vi "Arm Loop.vi"(8 "error in (no error)":errorcluster) -> ()   [LabVIEW 2012]
uses:
  Robot Global Data.vi
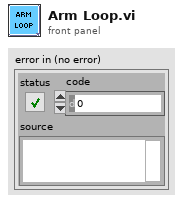
[diagram p1: front panel]
types:
  T1 = typedef "WPI_DriverStationRobotMode2.ctl" = enum16{"Autonomous Disabled", "Autonomous Enabled", "Teleop Disabled", "Teleop Enabled", "Timeout", "Finish", "Test Disabled", "Test Enabled"}
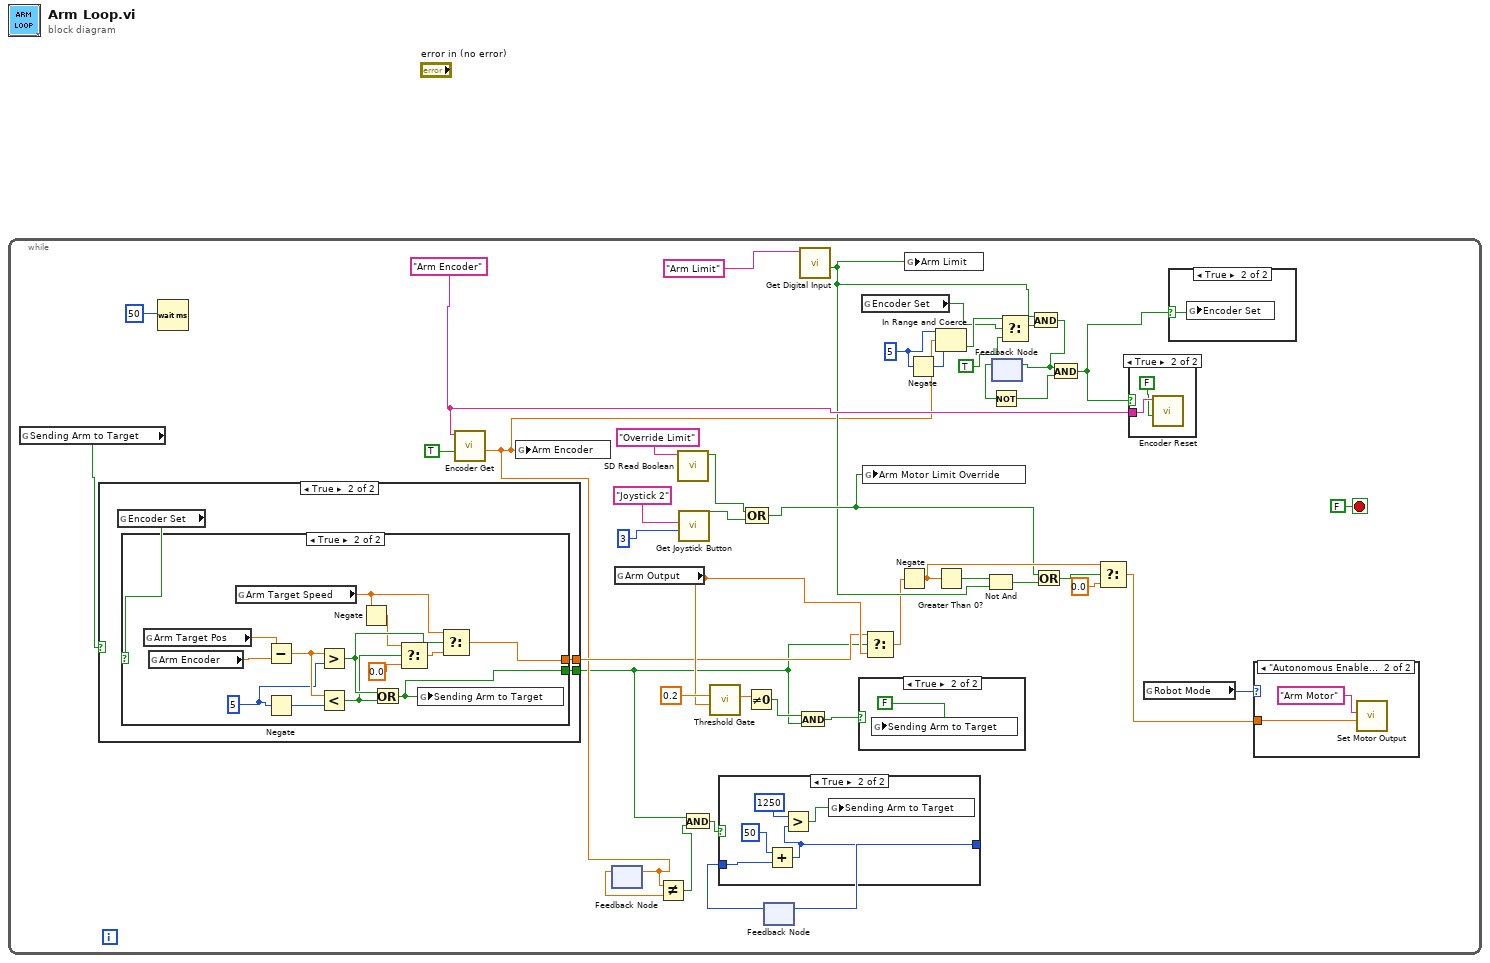
[diagram p0: block diagram]
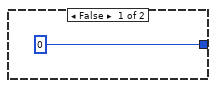
[diagram p2: hidden frame]
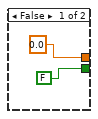
[diagram p5: hidden frame]
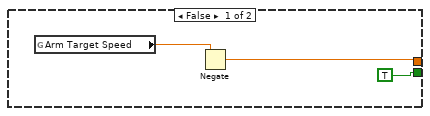
[diagram p6: hidden frame]
diagram:
  n1 = while {
    stop <- FALSE stop-if-true
    w26 = 5
    w29 = "Arm Encoder"
    n2 = global read "Robot Global Data.vi" "Sending Arm to Target"() -> (w16:bool)
    n3 = case shown="True" w16 {
      tunnel: [FALSE w57] -> w3
      tunnel: [0.0 w56] -> w12
      frame False {
      }
      frame True {
        n4 = global read "Robot Global Data.vi" "Encoder Set"() -> (w58:bool)
        n5 = case shown="True" w58 {
          tunnel: [TRUE w62] -> w57
          tunnel: [w60 w63] -> w56
          frame False {
            n6 = global read "Robot Global Data.vi" "Arm Target Speed"() -> (w61:dbl)
            n7 = Negate(x=w61) -> (-x=w60:dbl)
          }
          frame True {
            w66 = 5
            n8 = global read "Robot Global Data.vi" "Arm Target Pos"() -> (w67:dbl)
            n9 = global read "Robot Global Data.vi" "Arm Encoder"() -> (w68:dbl)
            n10 = global read "Robot Global Data.vi" "Arm Target Speed"() -> (w64:dbl)
            n11 = Subtract(x=w67, y=w68) -> (x-y=w74:dbl)
            n12 = Negate(x=w66) -> (-x=w73:i32)
            n13 = Greater?(x=w74, y=w66) -> (0:w71:bool)
            n14 = Less?(x=w74, y=w73) -> (x < y?=w69:bool)
            n15 = Negate(x=w64) -> (-x=w65:dbl)
            n16 = Or(x=w71, y=w69) -> (x .or. y?=w62:bool)
            n17 = Select(t=w65, s=w69, f=0.0) -> (s? t:f=w70:dbl)
            n18 = global write "Robot Global Data.vi" "Sending Arm to Target"(w62) -> ()
            n19 = Select(t=w64, s=w71, f=w70) -> (s? t:f=w63:dbl)
          }
        }
      }
    }
    n20 = Wait (ms)(milliseconds to wait=50) -> ()  [unwired: 1 out]
    n21 = call "Encoder Get.vi"("Use in Simulator (F)"=TRUE, "refnum name"=w29) -> ("Distance"=w7:dbl)  [unwired: 9 in]
    n22 = global write "Robot Global Data.vi" "Arm Encoder"(w7) -> ()
    n23 = feedback #1() -> (w6:dbl)  [unwired: 1 in]
    n24 = feedback-in #1(w7) -> ()
    n25 = global read "Robot Global Data.vi" "Arm Output"() -> (w13:dbl)
    n26 = Not Equal?(x=w7, y=w6) -> (x != y?=w2:bool)
    n27 = call <vilib>:"SD Read Boolean.vi"("Name"="Override Limit") -> ("Boolean"=w37:bool)  [unwired: 8 in, 2 out]
    n28 = call "Get Joystick Button.vi"("Button #"=3, "Joystick RefNum"="Joystick 2") -> ("Value"=w28:bool)  [unwired: 9 in]
    n29 = And(x=w3, y=w2) -> (x .and. y?=w1:bool)
    n30 = call "Threshold Gate.vi"("Value"=w13, "Threshold"=0.2) -> ("Output"=w17:dbl)  [unwired: 9 in]
    n31 = Compound Arithmetic op=OR(w37, w28) -> (w27:bool)
    n32 = Not Equal To 0?(x=w17) -> (x != 0?=w15:bool)
    n33 = feedback #2() -> (w5:i32)  [unwired: 1 in]
    n34 = case shown="True" w1 {
      tunnel: w5 -> [_ w50]
      tunnel: [0 w48] -> w4
      frame False {
      }
      frame True {
        n35 = Add(x=50, y=w50) -> (x+y=w48:i32)
        n36 = Greater?(x=1250, y=w48) -> (0:w46:bool)
        n37 = global write "Robot Global Data.vi" "Sending Arm to Target"(w46) -> ()
      }
    }
    n38 = feedback-in #2(w4) -> ()
    n39 = And(x=w15, y=w3) -> (x .and. y?=w11:bool)
    n40 = call "Get Digital Input.vi"("DigitalInput Refnum"="Arm Limit") -> ("Value"=w24:bool)  [unwired: 10 in]
    n41 = case shown="True" w11 {
      frame False {
      }
      frame True {
        n42 = global write "Robot Global Data.vi" "Sending Arm to Target"(FALSE) -> ()
      }
    }
    n43 = global read "Robot Global Data.vi" "Encoder Set"() -> (w19:bool)
    n44 = global write "Robot Global Data.vi" "Arm Motor Limit Override"(w27) -> ()
    n45 = Select(t=w12, s=w3, f=w13) -> (s? t:f=w14:dbl)
    n46 = Negate(x=w14) -> (-x=w36:dbl)
    n47 = global write "Robot Global Data.vi" "Arm Limit"(w24) -> ()
    n48 = Negate(x=w26) -> (-x=w25:i32)
    n49 = In Range and Coerce(upper limit=w26, x=w7, lower limit=w25) -> (In Range?=w20:bool)  [unwired: 1 out]
    n50 = Greater Than 0?(x=w36) -> (x > 0?=w34:bool)
    n51 = Not And(1:w24, 2:w34) -> (0:w32:bool)
    n52 = feedback #3() -> (w41:bool)  [unwired: 1 in]
    n53 = Not(x=w41) -> (.not. x?=w42:bool)
    n54 = Select(t=w20, s=w19, f=TRUE) -> (s? t:f=w23:bool)
    n55 = And(x=w24, y=w23) -> (x .and. y?=w22:bool)
    n56 = feedback-in #3(w22) -> ()
    n57 = Or(x=w27, y=w32) -> (x .or. y?=w33:bool)
    n58 = And(x=w22, y=w42) -> (x .and. y?=w8:bool)
    n59 = Select(t=w36, s=w33, f=0.0) -> (s? t:f=w31:dbl)
    n60 = case shown="True" w8 {
      tunnel: w29 -> [_ w52]
      frame False {
      }
      frame True {
        n61 = call "Encoder Reset.vi"("Use in Simulator (F)"=FALSE, "refnum name"=w52) -> ()  [unwired: 10 in]
      }
    }
    n62 = global read "Robot Global Data.vi" "Robot Mode"() -> (w30:T1)
    n63 = case shown="True" w8 {
      selector: w8 -> [_ w75]
      frame False {
      }
      frame True {
        n64 = global write "Robot Global Data.vi" "Encoder Set"(w75) -> ()
      }
    }
    n65 = case shown="\"Autonomous Enabled\", \"Teleop Enabled\", \"Test Enabled\"" w30 {
      tunnel: w31 -> [_ w77]
      frame Default {
      }
      frame "Autonomous Enabled", "Teleop Enabled", "Test Enabled" {
        n66 = call "Set Motor Output.vi"("Output"=w77, "Motor RefNum"="Arm Motor") -> ()  [unwired: 10 in]
      }
    }
  }
